vi "OpenWindowsExplorer.vi"(0 "Directory or File":path, 2 "Select Directory? (F: Open Directory)":bool, 5 "error in (no error)":errorcluster) -> (19 "error out":errorcluster)   [LabVIEW 2020]
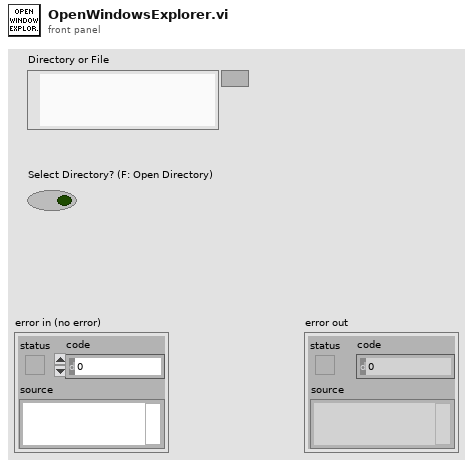
[diagram p1: front panel]
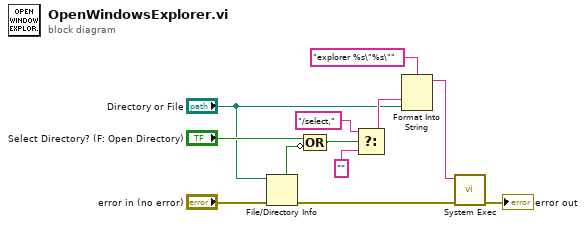
[diagram p0: block diagram]
diagram:
  n1 = File/Directory Info(path="Directory or File", error in="error in (no error)") -> (directory=w9:bool, error out=w7:errorcluster)  [unwired: 5 out]
  n2 = Compound Arithmetic op=OR("Select Directory? (F: Open Directory)", invert w9) -> (w5:bool)
  n3 = Select(t="/select," ("format string"), s=w5, f="") -> (s? t:f=w4:string)
  n4 = Format Into String(format string="explorer %s\"%s\"", w4, "Directory or File") -> (resulting string=w11:string)  [unwired: 2 in, 1 out]
  n5 = call <vilib>:"System Exec.vi"("error in (no error)"=w7, "command line"=w11) -> ("error out"=→"error out":errorcluster)  [unwired: 6 in, 3 out]
